vi "Read Client ID.vi"(8 "error in":errorcluster, 11 "Launch Client in":refnum<class "Launch Client.lvclass">) -> (0 "error out":errorcluster, 2 "Client ID":string, 3 "Launch Client out":refnum<class "Launch Client.lvclass">)   [LabVIEW 2014, in "Launch Client.lvclass"]
uses:
  Launch Client.lvclass
  Architecture/Classes/Topic_class/Topic.lvclass
  Launch Client.lvclass/Launch Client.ctl
panel:
  in  "Topic in":refnum<class "Topic.lvclass">
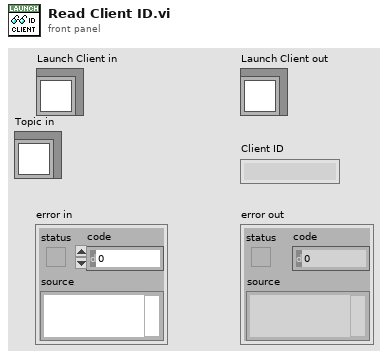
[diagram p1: front panel]
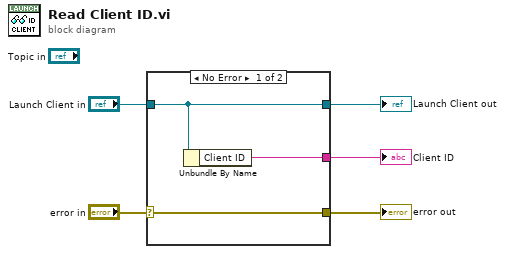
[diagram p0: block diagram]
diagram:
  n1 = case shown="No Error" "error in" {
    selector: "error in" -> [w8 w9]
    tunnel: [w8 w9] -> w4
    tunnel: [w7 w10] -> w2
    tunnel: "Launch Client in" -> [w7 w10]
    tunnel: [w6 _] -> w1
    frame No Error {
      n2 = Unbundle By Name(w7) -> ("Client ID"=w6:string)
    }
    frame Error {
    }
  }
  "error out" <- w4
  "Launch Client out" <- w2
  "Client ID" <- w1
